vi "ProgramControlSafetyMode.vi"(0 "Front Panel Controls in":T2, 5 "Safety Status":T1) -> (14 "Front Panel Controls out":T2)   [LabVIEW 2019, in "Universal Robot.lvclass"]
uses:
  Universal Robot.lvclass
  ProgramControlFPControls.ctl
  SafetyStatus.ctl
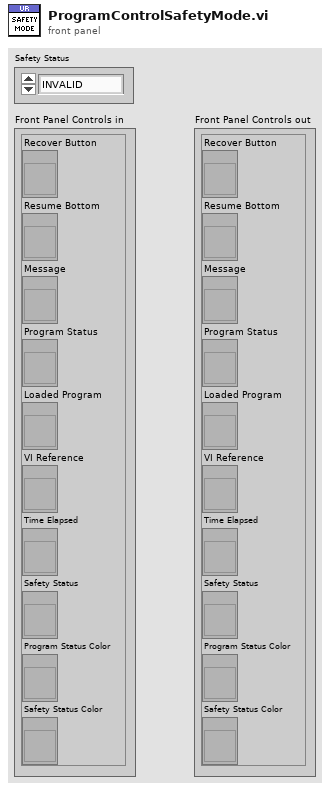
[diagram p1: front panel]
types:
  T1 = typedef "Universal Robot.lvclass/SafetyStatus.ctl" = enum16{"INVALID", "NORMAL", "REDUCED", "PROTECTIVE_STOP", "RECOVERY", "SAFEGUARD_STOP", "SYSTEM_EMERGENCY_STOP", "ROBOT_EMERGENCY_STOP", "VIOLATION", "FAULT", "AUTOMATIC_MODE_SAFEGAURD_STOP", "SYSTEM_THREE_POSITION_ENABLING_STOP"}
  T2 = typedef "Universal Robot.lvclass/ProgramControlFPControls.ctl" = cluster{"Recover Button":refnum<vi>, "Resume Bottom":refnum<vi>, "Message":refnum<vi>, "Program Status":refnum<vi>, "Loaded Program":refnum<vi>, "VI Reference":refnum<vi>, "Time Elapsed":refnum<vi>, "Safety Status":refnum<vi>, "Program Status Color":refnum<vi>, "Safety Status Color":refnum<vi>}
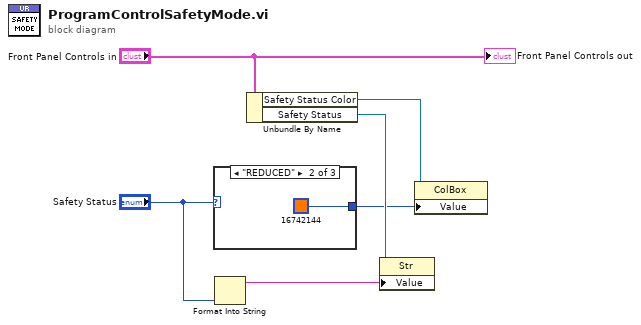
[diagram p0: block diagram]
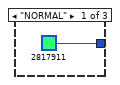
[diagram p2: hidden frame]
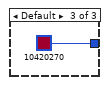
[diagram p3: hidden frame]
diagram:
  n1 = case shown="\"REDUCED\"" "Safety Status" {
    tunnel: [u32 2817911 u32 16742144 u32 10420270] -> w1
    frame "NORMAL" {
    }
    frame "REDUCED" {
    }
    frame Default {
    }
  }
  n2 = Format Into String("Safety Status") -> (resulting string=w3:string)  [unwired: 3 in, 1 out]
  n3 = Unbundle By Name("Front Panel Controls in") -> ("Safety Status Color"=w2:refnum<vi>, "Safety Status"=w5:refnum<vi>)
  n4 = property class="Str"(reference=w5, "Value"=w3) -> ()  [unwired: 1 in, 2 out]
  n5 = property class="ColBox"(reference=w2, "Value"=w1) -> ()  [unwired: 1 in, 2 out]
  "Front Panel Controls out" <- "Front Panel Controls in"
